vi "test_ICLshutdown.vi"(8 "error in":errorcluster) -> (0 "error out":errorcluster)   [LabVIEW 2020, in "horiba.test.lvlib"]
doc: "_____\nCreated using DQMH Event Scripter 7.0.1.1316."
uses:
  horiba.test.lvlib
  Classes/DeviceManager/DeviceManager.lvlib
  <vilib>/addons/_JKI Toolkits/Caraya/classes/Assert/Assert True.vi
  <vilib>/addons/_JKI Toolkits/Caraya/classes/Assert/Assert Not Error.vi
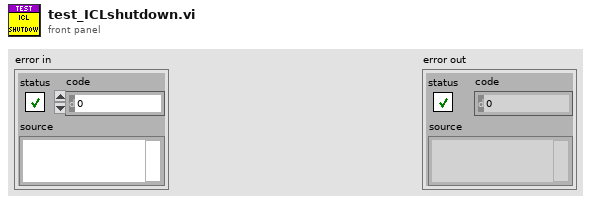
[diagram p1: front panel]
types:
  T1 = typedef "horiba.lvlib/DeviceManager.lvlib/Broadcast Events--cluster.ctl" = cluster{"Module Did Init":refnum<user-event>, "Status Updated":refnum<user-event>, "Error Reported":refnum<user-event>, "Module Did Stop":refnum<user-event>, "Update Module Execution Status":refnum<user-event>, "iclIsRunning":refnum<user-event>, "websocketConnectionOpened":refnum<user-event>, "devicesDiscovered":refnum<user-event>}
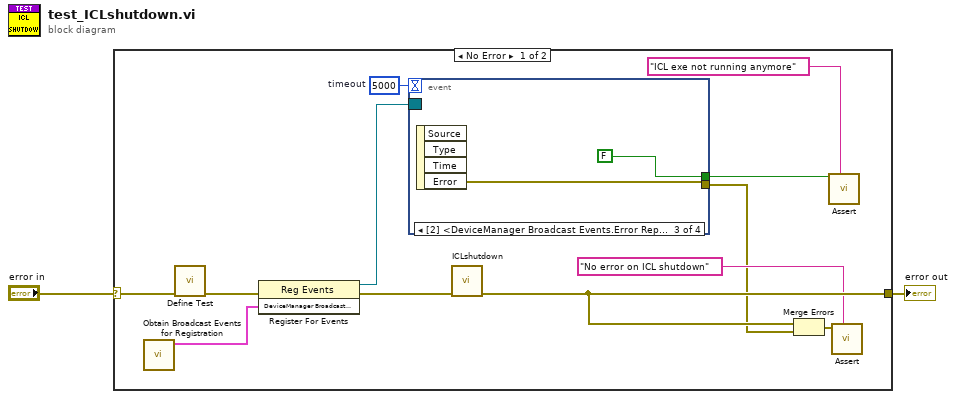
[diagram p0: block diagram]
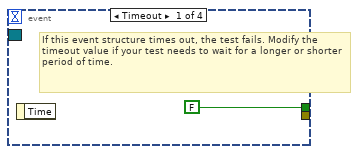
[diagram p2: hidden frame]
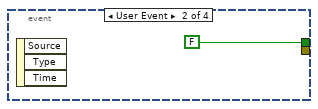
[diagram p3: hidden frame]
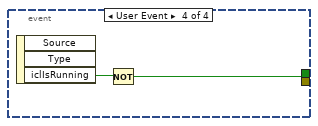
[diagram p4: hidden frame]
diagram:
  n1 = case shown="No Error" "error in" {
    selector: "error in" -> [w14 w21]
    tunnel: [w8 w21] -> w1
    frame No Error {
      w10 = 5000  # timeout
      n2 = call "Obtain Broadcast Events for Registration.vi"() -> ("DeviceManager Broadcast Events"=w12:T1)  [unwired: 9 in, 2 out]
      n3 = call <vilib>:"Define Test.vi"("error in (no error)"=w14) -> ("error out"=w3:errorcluster)  [unwired: 9 in, 1 out]
      n4 = register-events(error in=w3, w12) -> (reference out=w11:refnum<event-registration>, error out=w13:errorcluster)  [unwired: 1 in]
      n5 = event shown="[2] <DeviceManager Broadcast Events.Error Reported>: User Event" {
        selector: w11 -> [_ _ _ _]
        dyn-events: _ -> [_ _ _ _]
        timeout: w10 -> [_ _ _ _]
        tunnel: [FALSE FALSE FALSE w19] -> w6
        tunnel: [_ _ w17 _] -> w4
        event Timeout {
          # "If this event structure times out, the test fails. Modify the timeout value if your test needs to wait for a longer or shorter period of time."
          n6 = event-data() -> ()  [unwired: 1 in, 1 out]
        }
        event User Event {
          n7 = event-data() -> ()  [unwired: 1 in, 3 out]
        }
        event User Event {
          n8 = event-data() -> ("Error"=w17:errorcluster)  [unwired: 1 in, 3 out]
        }
        event User Event {
          n9 = event-data() -> ("iclIsRunning"=w20:bool)  [unwired: 1 in, 2 out]
          n10 = Not(x=w20) -> (.not. x?=w19:bool)
        }
      }
      n11 = call "ICLshutdown.vi"("error in"=w13) -> ("error out"=w8:errorcluster)  [unwired: 10 in]
      n12 = Merge Errors(w8, w4) -> (w5:errorcluster)
      n13 = call-poly <vilib>:"Assert.vi"("Label"="ICL exe not running anymore", "True?"=w6) -> ()  [unwired: 8 in, 2 out]
      n14 = call-poly <vilib>:"Assert.vi"("Label"="No error on ICL shutdown", "Not Error?"=w5) -> ()  [unwired: 8 in, 2 out]
    }
    frame Error {
    }
  }
  "error out" <- w1
